vi "Destroy User Events.vi"(11 "UI Template in":refnum<class "Home.lvclass">) -> (3 "UI Template out":refnum<class "Home.lvclass">)   [LabVIEW 2024, in "Home.lvlib" / "Home.lvclass"]
uses:
  Home.lvclass
  Home.lvclass/Home.ctl
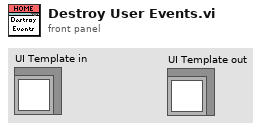
[diagram p1: front panel]
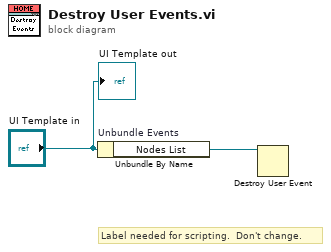
[diagram p0: block diagram]
diagram:
  # "Label needed for scripting.  Don't change."
  n1 = Unbundle By Name "Unbundle Events"("UI Template in") -> ("Nodes List"=w2:refnum<user-event>)
  n2 = Destroy User Event(user event=w2) -> ()  [unwired: 1 in, 1 out]
  "UI Template out" <- "UI Template in"
